vi "Agilent 681x Standard Triggered Output.vi"() -> ()   [LabVIEW 2019]
doc: "Demonstrates how to use the output triggering system to change output voltage with a trigger."
uses:
  <instrlib>/Agilent 681x Series/Agilent 681x Series.lvlib
panel:
  in  "Pulse Characteristic Value (50)":dbl=50.0 format="%#.4g"
  in  "Pulse Characteristic (0: Duty Cycle)":u16(ring) items=["Duty Cycle", "Pulse Width"]
  in  "Period (0.0333 s)":dbl=0.03333 format="%#.4g"
  in  "Pulse Count (1)":dbl=1.0 format="%#.4g"
  in  "Trigger Delay (0 s)":dbl format="%#.5g"
  in  "Voltage Mode (0: Fix)":u16(ring) items=["Fixed", "Step", "Pulse", "List"]
  in  "Voltage Amplitude (1.0 V)":dbl=1.0 format="%#.4g"
  in  "Triggered Voltage Amplitude (1.0 V)":dbl=1.0 format="%#.4g"
  in  "Serial Configuration":T1={"Baud Rate"=9600, "Parity"=0, "Data Bits"=8} {"Data Bits" items=["7"=7, "8"=8]; "Parity" items=["None", "Odd", "Even", "Mark", "Space"]; "Baud Rate" items=["300"=300, "600"=600, "1200"=1200, "2400"=2400, "4800"=4800, "9600"=9600]}
  in  "VISA resource name":refnum<visa-resource-name>
  # "VI para definir:\n    1) amplitude da tensão de saída da fonte  (voltage amplitude)\n    2) modo de tensão (fixo, degrau, pulso, lista)  (voltage mode)\n    3) amplitude da tensão a ser \"triggada\" (triggered voltage amplitude)\n    4) delay para aplicar a tensão a ser \"triggada\" (trigger delay) \n    5) período da onda \"triggada\" (period)\n    6) largura do pulso (pulse width) ou duty cycle onde a tensão \"triggada\" ficará ativada (pulse characteristic value)\n    7) característica do pulso (largura em s ou  duty cycle em %)  (pulse characteristic)"
  # "(c) 2008-2021 National Instruments Corp.  ALL RIGHTS RESERVED."
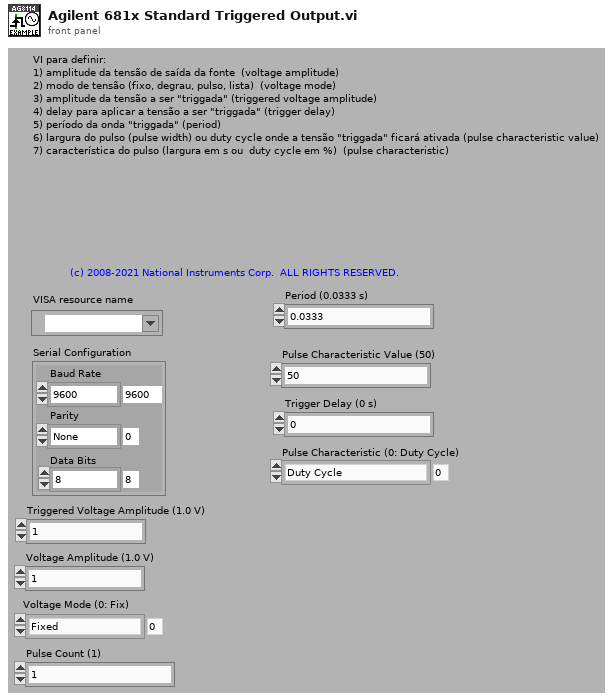
[diagram p1: front panel]
types:
  T1 = cluster{"Baud Rate":u32, "Parity":u16, "Data Bits":u16}
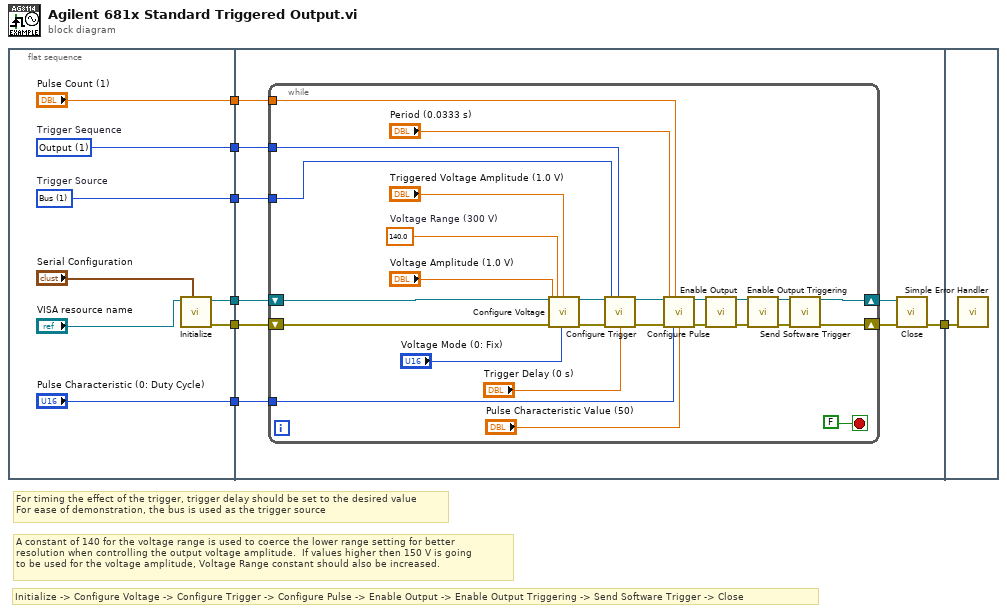
[diagram p0: block diagram]
diagram:
  # "For timing the effect of the trigger, trigger delay should be set to the desired value\nFor ease of demonstration, the bus is used as the trigger source"
  # "Initialize -> Configure Voltage -> Configure Trigger -> Configure Pulse -> Enable Output -> Enable Output Triggering -> Send Software Trigger -> Close"
  # "A constant of 140 for the voltage range is used to coerce the lower range setting for better\nresolution when controlling the output voltage amplitude.  If values higher then 150 V is going\nto be used for the voltage amplitude, Voltage Range constant should also be increased."
  n1 = flat-sequence {
    tunnel: ["Pulse Count (1)"] -> w7
    tunnel: ["Pulse Characteristic (0: Duty Cycle)"] -> w6
    tunnel: [w11] -> w5
    tunnel: [w10] -> w4
    tunnel: [w9] -> w3
    tunnel: [w8] -> w2
    tunnel: w7 -> [w22]
    tunnel: w6 -> [w21]
    tunnel: w5 -> [w20]
    tunnel: w4 -> [w19]
    tunnel: w3 -> [w18]
    tunnel: w2 -> [w17]
    tunnel: [w16] -> w1
    tunnel: w1 -> [w51]
    frame #0 {
      w10 = 1 items=["Immediate", "Bus", "External", "Phase", "Trigger Out"]  # Trigger Source
      w11 = 1 items=["Output"=1, "Synchronous Source"=2, "Measurement"=3]  # Trigger Sequence
      n2 = call <instrlib>:"Initialize.vi"("Serial Configuration"="Serial Configuration", "VISA resource name"="VISA resource name") -> ("error out"=w8:errorcluster, "VISA resource name out"=w9:refnum<visa-resource-name>)  [unwired: 8 in]
    }
    frame #1 {
      n3 = while {
        tunnel: w22 -> [w38]
        tunnel: w21 -> [w37]
        tunnel: w20 -> [w36]
        tunnel: w19 -> [w35]
        shift-right: [w50] -> w24
        shift-left: w18 -> [w34]
        shift-right: [w49] -> w23
        shift-left: w17 -> [w33]
        stop <- FALSE stop-if-true
        w28 = 140.0  # Voltage Range (300 V)
        n4 = call <instrlib>:"Configure Voltage.vi"("VISA resource name"=w34, "Triggered Voltage Amplitude (1.0 V)"="Triggered Voltage Amplitude (1.0 V)", "Voltage Range (300 V)"=w28, "Voltage Amplitude (1.0 V)"="Voltage Amplitude (1.0 V)", "Voltage Mode (0: Fix)"="Voltage Mode (0: Fix)", "error in (no error)"=w33) -> ("VISA resource name out"=w48:refnum<visa-resource-name>, "error out"=w47:errorcluster)  [unwired: 8 in]
        n5 = call <instrlib>:"Configure Trigger.vi"("VISA resource name"=w48, "Trigger Sequence (1: Output 1)"=w36, "Trigger Source (0: Immediate)"=w35, "error in (no error)"=w47, "Trigger Delay (0 s)"="Trigger Delay (0 s)") -> ("VISA resource name out"=w42:refnum<visa-resource-name>, "error out"=w41:errorcluster)  [unwired: 9 in]
        n6 = call <instrlib>:"Configure Pulse.vi"("VISA resource name"=w42, "Pulse Count (1)"=w38, "Period (0.0333 s)"="Period (0.0333 s)", "error in (no error)"=w41, "Pulse Characteristic (0: Duty Cycle)"=w37, "Pulse Characteristic Value (50)"="Pulse Characteristic Value (50)") -> ("VISA resource name out"=w44:refnum<visa-resource-name>, "error out"=w43:errorcluster)  [unwired: 8 in]
        n7 = call <instrlib>:"Enable Output.vi"("VISA resource name"=w44, "error in (no error)"=w43) -> ("VISA resource name out"=w39:refnum<visa-resource-name>, "error out"=w40:errorcluster)  [unwired: 12 in]
        n8 = call <instrlib>:"Enable Output Triggering.vi"("VISA resource name"=w39, "error in (no error)"=w40) -> ("VISA resource name out"=w45:refnum<visa-resource-name>, "error out"=w46:errorcluster)  [unwired: 12 in]
        n9 = call <instrlib>:"Send Software Trigger.vi"("VISA resource name"=w45, "error in (no error)"=w46) -> ("VISA resource name out"=w50:refnum<visa-resource-name>, "error out"=w49:errorcluster)  [unwired: 12 in]
      }
      n10 = call <instrlib>:"Close.vi"("error in (no error)"=w23, "VISA resource name"=w24) -> ("error out"=w16:errorcluster)  [unwired: 9 in]
    }
    frame #2 {
      n11 = call <vilib>:"Simple Error Handler.vi"("error in (no error)"=w51) -> ()  [unwired: 4 in, 5 out]
    }
  }
